vi "TDT Test Marker Read.vi"() -> ()   [LabVIEW 2020]
uses:
  Typedefs/TDT-Output source.ctl
  Typedefs/TDT-Device ID.ctl
  Utility VIs/Controls/Utilities-Wait.vi/89bc9713-8f2c-40bd-a11f-1c800a437687.vi
  <vilib>/Utility/High Resolution Polling Wait.vi
panel:
  out "GetTagVal":sgl
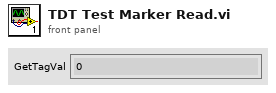
[diagram p1: front panel]
types:
  T1 = typedef "TDT-Output source.ctl" = cluster{"Device":T2, "Num":i32}
  T2 = typedef "TDT-Device ID.ctl" = enum16{"None", "PA5", "RP2", "RL2", "RA16", "RV8", "RX5", "RX6", "RX7", "RX8", "RZ2", "RZ5", "RZ6"}
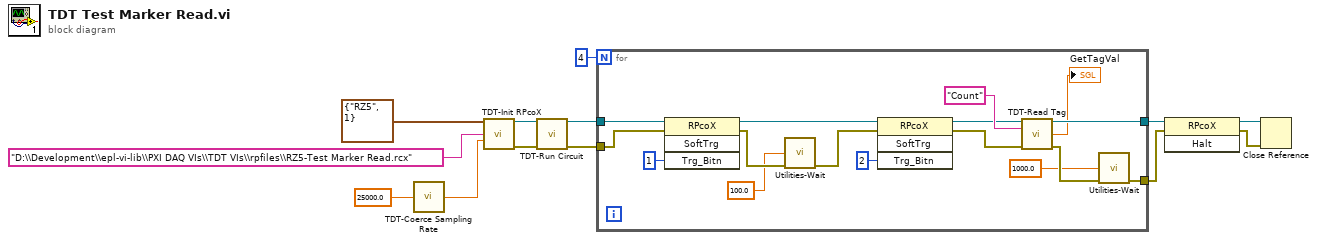
[diagram p0: block diagram]
diagram:
  n1 = call "TDT-Coerce Sampling Rate.vi"("Fs (Hz)"=25000.0 ("AO Sampling Rate (Hz)")) -> ("Coerced"=w10:dbl)
  n2 = call "TDT-Init RPcoX.vi"("Output"=T1 {"Device"=enum."RZ5", "Num"=1}, "RPfilename"="D:\\Development\\epl-vi-lib\\PXI DAQ VIs\\TDT VIs\\rpfiles\\RZ5-Test Marker Read.rcx", "Sampling rate (Hz)"=w10) -> ("RPcoX"=w4:refnum<k7>, "error out"=w1:errorcluster)  [unwired: 11 in]
  n3 = call "TDT-Run Circuit.vi"("RPcoX"=w4, "error in (no error)"=w1) -> ("RPcoX out"=w3:refnum<k7>, "error out"=w2:errorcluster)  [unwired: 12 in]
  n4 = for {
    N: 4 -> [_]
    tunnel: w3 -> [w28]
    tunnel: w2 -> [w27]
    tunnel: [w16] -> w6
    tunnel: [w15] -> w5
    n5 = invoke class="RPcoX" method="SoftTrg"(reference=w28, error in=w27, "Trg_Bitn"=1) -> (reference out=w22:refnum<k7>, error out=w26:errorcluster)  [unwired: 1 in, 2 out]
    n6 = call "Utilities-Wait.vi"("milliseconds to wait"=100.0, "error in (no error)"=w26) -> ("error out"=w21:errorcluster)  [unwired: 13 in]
    n7 = invoke class="RPcoX" method="SoftTrg"(reference=w22, error in=w21, "Trg_Bitn"=2) -> (reference out=w20:refnum<k7>, error out=w19:errorcluster)  [unwired: 1 in, 2 out]
    n8 = call "TDT-Read Tag.vi"("RPcox"=w20, "Name"="Count", "error in"=w19) -> ("RPcox Out"=w16:refnum<k7>, "GetTagVal"=→"GetTagVal":sgl, "error out"=w18:errorcluster)  [unwired: 10 in]
    n9 = call "Utilities-Wait.vi"("milliseconds to wait"=1000.0, "error in (no error)"=w18) -> ("error out"=w15:errorcluster)  [unwired: 13 in]
  }
  n10 = invoke class="RPcoX" method="Halt"(reference=w6, error in=w5) -> (reference out=w8:refnum<k7>, error out=w7:errorcluster)  [unwired: 1 in, 1 out]
  n11 = Close Reference(reference=w8, error in (no error)=w7) -> ()  [unwired: 1 out]
